vi "MT Demodulate Offset PSK.vi"(0 "input complex waveform":T4={"t0"=0.0, "dt"=1.0, "Y"=[]} {"Y" format="%.3f"; "dt" format="%^.2e"; "t0" format="%.4f"}, 5 "Offset PSK system parameters":T3={"samples per symbol (16)"=16, "symbol map"=[], "differential Offset PSK"=enum."disable"} {"symbol map" format="%.3f"}, 7 "matched filter coefficients":dbl[](array[numeric]) format="%.2f", 9 "synchronization parameters":T2 {"sync sequence" format="%.2f"}, 11 "error in (no error)":errorcluster, 12 "pulse shaping filter coefficients":dbl[](array[numeric]) format="%.2f", 13 "reset? (T)":bool=TRUE) -> (4 "recovered complex waveform":T4 {"Y" format="%.3f"; "dt" format="%^.2e"; "t0" format="%.4f"}, 6 "output bit stream":i8[](array[numeric]), 8 "measurements":T1 {"phase offset (deg)" format="%.2f"; "frequency drift (Hz)" format="%.2f"; "frequency offset (Hz)" format="%.2f"}, 10 "sync found index (symbols)":dbl format="%.4f", 15 "error out":errorcluster)   [LabVIEW 2020, in "niDMT.lvlib"]
doc: "Demodulates a offset PSK-modulated complex baseband waveform and returns the time-aligned oversampled complex waveform, the demodulated bit stream, and measurement results obtained during demodulation. This VI attempts to remove carrier and phase offset by locking to the carrier signal. \n\nNOTE: Offset mode is only supported for 4-PSK (OQPSK), and use of the offset mode requires some form of band-limiting filtration. Raised cosine and root raised cosine are the only valid filter types for OQPSK demodulation. Demodulator locking performance degrades with alpha values <0.3 in the raised cosine or root raised cosine filter design."
uses:
  <vilib>/addons/Modulation/niDMT.lvlib
  <vilib>/addons/Modulation/Analog/controls/Complex Data Waveform.ctl
  <vilib>/addons/Modulation/Digital/Support/Controls/Offset PSK System Parameters.ctl
  <vilib>/addons/Modulation/Analog/MT Resample (Complex Cluster).vi
  <vilib>/addons/Modulation/Digital/Support/Common/mod_Apply Frequency Offset (Internal).vi
  <vilib>/addons/Modulation/Analog/support/Validators/mod_Fractional Resample Validate.vi
  <vilib>/addons/Modulation/Analog/support/Validators/mod_Check Flush State.vi
  <vilib>/addons/Modulation/Analog/support/mod_FractionalResampler.vi
  <vilib>/addons/Modulation/Analog/support/mod_Integer Rate Interpolation.vi
  <vilib>/addons/Modulation/Analog/support/Validators/mod_Validate Complex Waveform.vi
  <vilib>/addons/Modulation/Analog/support/mod_PerformResampling.vi
  <vilib>/addons/Modulation/Analog/support/Validators/mod_WFErrorHandler.vi
  <vilib>/addons/Modulation/Digital/Support/Common/mod_Truncate FIR Filter (complex).vi
  <vilib>/Utility/error.llb/Error Cluster From Error Code.vi
  <vilib>/addons/Modulation/Analog/support/mod_Resampling Factors.vi
  <vilib>/addons/Modulation/Analog/support/mod_ResamplingFilter.vi
  <vilib>/addons/Modulation/Analog/support/mod_Generate Integer Interpolation Filter.vi
  <vilib>/addons/Modulation/niAMT.lvlib
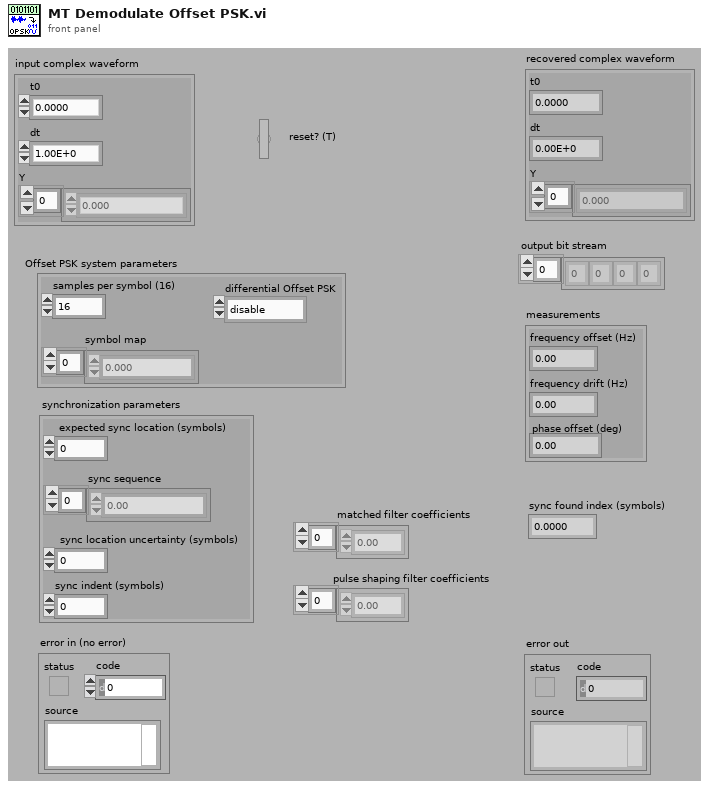
[diagram p1: front panel]
types:
  T1 = cluster{"frequency offset (Hz)":dbl, "frequency drift (Hz)":dbl, "phase offset (deg)":dbl}
  T2 = cluster{"expected sync location (symbols)":i32, "sync sequence":cdb[], "sync location uncertainty (symbols)":i32, "sync indent (symbols)":i32}
  T3 = typedef "niDMT.lvlib/Offset PSK System Parameters.ctl" = cluster{"samples per symbol (16)":i32, "symbol map":cdb[], "differential Offset PSK":enum16{"disable", "enable"}}
  T4 = typedef "niAMT.lvlib/Complex Data Waveform.ctl" = cluster{"t0":dbl, "dt":dbl, "Y":cdb[]}
  T5 = cluster{dbl, "Frequency Drift, Hz":dbl, "Phase Error Estimate, rads":dbl}
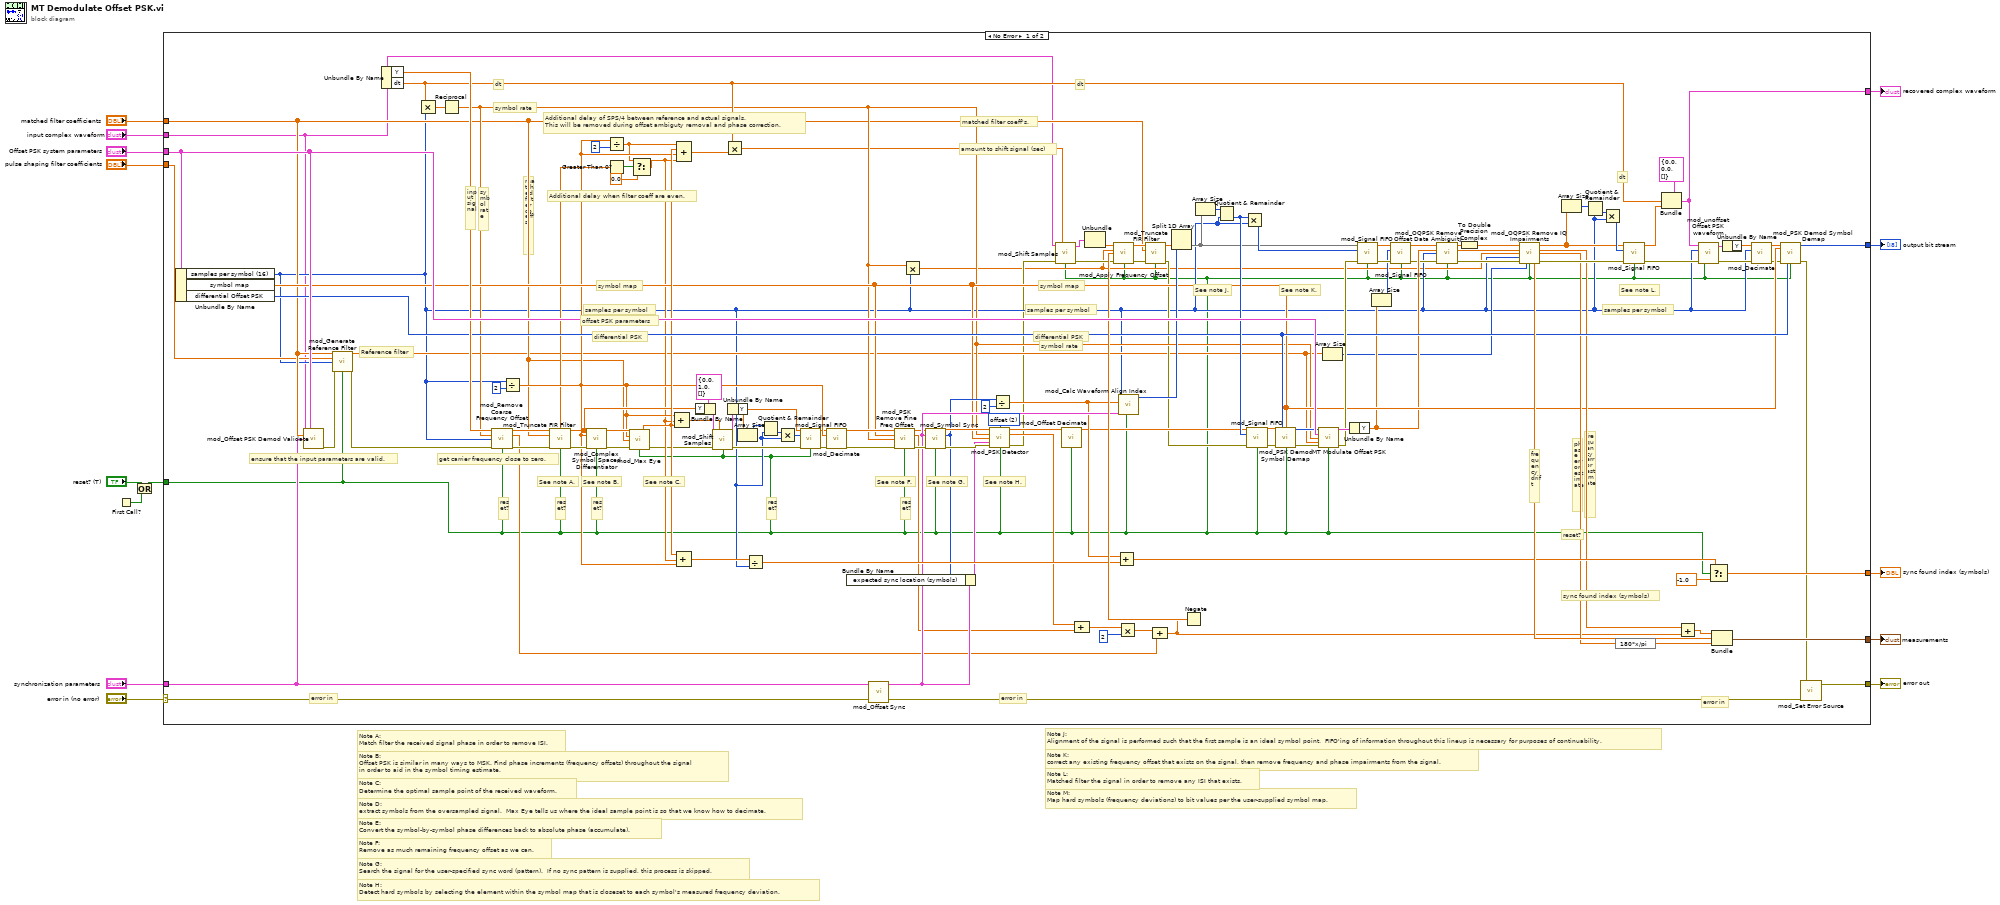
[diagram p0: block diagram]
diagram:
  # "Note E:\nConvert the symbol-by-symbol phase differences back to absolute phase (accumulate)."
  # "Note B:\nOffset PSK is similar in many ways to MSK. Find phase increments (frequency offsets) throughout the signal\nin order to aid in the symbol timing estimate."
  # "Note M:\nMap hard symbols (frequency deviations) to bit values per the user-supplied symbol map."
  # "Note J:\nAlignment of the signal is performed such that the first sample is an ideal symbol point.  FIFO'ing of information throughout this lineup is necessary for purposes of continuability."
  # "Note G:\nSearch the signal for the user-specified sync word (pattern).  If no sync pattern is supplied, this process is skipped."
  # "Note F:\nRemove as much remaining frequency offset as we can."
  # "Note D:\nextract symbols from the oversampled signal.  Max Eye tells us where the ideal sample point is so that we know how to decimate."
  # "Note C:\nDetermine the optimal sample point of the received waveform."
  # "Note A:\nMatch filter the received signal phase in order to remove ISI."
  # "Note H:\nDetect hard symbols by selecting the element within the symbol map that is closeset to each symbol's measured frequency deviation."
  # "Note K:\ncorrect any existing frequency offset that exists on the signal, then remove frequency and phase impairments from the signal."
  # "Note L:\nMatched filter the signal in order to remove any ISI that exists."
  n1 = First Call?() -> (First Call?: T/F=w5:bool)
  n2 = Or(x="reset? (T)", y=w5) -> (x .or. y?=w3:bool)
  n3 = case shown="No Error" "error in (no error)" {
    selector: "error in (no error)" -> [w136 w142]
    tunnel: w3 -> [w15 _]
    tunnel: "input complex waveform" -> [w19 _]
    tunnel: [w137 w142] -> w12
    tunnel: "matched filter coefficients" -> [w25 _]
    tunnel: [w64 _] -> w8
    tunnel: [w140 _] -> w11
    tunnel: [w89 _] -> w6
    tunnel: "Offset PSK system parameters" -> [w139 _]
    tunnel: "synchronization parameters" -> [w138 _]
    tunnel: [w141 _] -> w7
    tunnel: "pulse shaping filter coefficients" -> [w24 _]
    frame No Error {
      w54 = u16 2 items=["normal", "shifted", "offset"] ("PSK type")
      # "Additional delay when filter coeff are even."
      # "Additional delay of SPS/4 between reference and actual signals.\nThis will be removed during offset ambiguty removal and phase correction."
      # "Reference filter"
      # "samples per symbol"
      # "samples per symbol"
      # "dt"
      # "dt"
      # "dt"
      # "matched filter coeff's."
      # "symbol rate"
      # "offset PSK parameters"
      # "symbol map"
      # "symbol map"
      # "amount to shift signal (sec)"
      # "matched filter coeff's."
      # "input signal"
      # "symbol rate"
      # "differential PSK"
      # "differential PSK"
      # "samples per symbol"
      # "frequency error estimate"
      # "phase error estimate"
      # "frequency drift"
      # "reset?"
      # "sync found index (symbols)"
      # "reset?"
      # "reset?"
      # "reset?"
      # "reset?"
      # "reset?"
      # "error in"
      # "error in"
      # "error in"
      # "See note L."
      # "See note K."
      # "See note J."
      # "See note H."
      # "See note G."
      # "ensure that the input parameters are valid."
      # "See note A."
      # "See note B."
      # "get carrier frequency close to zero."
      # "See note C."
      # "See note F."
      # "symbol rate"
      n4 = Unbundle By Name(w139) -> ("samples per symbol (16)"=w22:i32, "symbol map"=w72:cdb[], "differential Offset PSK"=w86:enum16{"disable", "enable"})
      n5 = call <vilib>:"mod_Offset PSK Demod Validate.vi"("Input Complex Waveform"=w19, "PSK System Parameters"=w139, "Matched Filter Coefficients"=w25, "Synchronization Parameters"=w138) -> ("error out"=w21:errorcluster)  [unwired: 11 out]
      n6 = call <vilib>:"mod_Generate Reference Filter.vi"("matched filter coefficients"=w25, "pulse shaping filter coefficients"=w24, "samples per symbol (16)"=w22, "error in (no error)"=w21, "reset? (T)"=w15) -> ("reference filter coefficients"=w23:dbl[], "error out"=w20:errorcluster)  [unwired: 9 in]
      n7 = Unbundle By Name(w19) -> ("Y"=w113:cdb[], "dt"=w73:dbl)
      n8 = Multiply(x=w73, y=w22) -> (x*y=w134:dbl)
      n9 = Reciprocal(x=w134) -> (1/x=w71:dbl)
      n10 = call <vilib>:"mod_Remove Coarse Frequency Offset.vi"("Signal In"=w113, "Symbol Rate, Hz"=w71, "Samples Per Symbol (16)"=w22, "error in (no error)"=w20, "Reset? (T)"=w15) -> ("Signal Out"=w85:cdb[], "Freq Est, Hz"=w91:dbl, "error out"=w116:errorcluster)  [unwired: 8 out]
      n11 = Divide(x=w22, y=2) -> (x/y=w44:dbl)
      n12 = call-poly <vilib>:"mod_Truncate FIR Filter.vi"("Signal In"=w85, "Filter Coefficients"=w25, "error in (no error)"=w116, "Reset? (T)"=w15) -> ("Fractional Delay (samples)"=w41:dbl, "Signal Out"=w45:cdb[], "error out"=w115:errorcluster)  [unwired: 8 in, 1 out]
      n13 = call <vilib>:"mod_Complex Symbol Spaced Differentiator.vi"("Signal In"=w45, "Samples Per Symbol (16)"=w44, "error in (no error)"=w115, "Reset? (T)"=w15) -> ("Signal Out"=w112:cdb[], "error out"=w122:errorcluster)  [unwired: 10 out]
      n14 = Divide(x=w44, y=2) -> (x/y=w40:dbl)
      n15 = Greater Than 0?(x=w41) -> (x > 0?=w43:bool)
      n16 = call <vilib>:"mod_Max Eye.vi"("Signal In"=w112, "Samples Per Symbol (16)"=w44, "Filter Coefficients"=w25, "error in (no error)"=w122, "Reset? (T)"=w15) -> ("Waveform Alignment Offset"=w80:dbl, "error out"=w27:errorcluster)  [unwired: 6 in, 3 out]
      n17 = Select(t=w40, s=w43, f=0.0) -> (s? t:f=w39:dbl)
      n18 = Compound Arithmetic op=ADD(w44, w39, w80) -> (w28:dbl)
      n19 = Compound Arithmetic op=ADD(w80, w39, w44) -> (w114:dbl)
      n20 = Compound Arithmetic op=ADD(w40, w80, w44, w39) -> (w62:dbl)
      n21 = Bundle By Name(cluster=T4 {"t0"=0.0, "dt"=1.0, "Y"=[]} ("Input Complex Waveform"), "Y"=w45) -> (w29:T4)
      n22 = call <vilib>:"mod_Shift Samples.vi"("Input Complex Waveform"=w29, "Initial Sample Offset, sec"=w28, "error in (no error)"=w27, "Reset? (T)"=w15) -> ("Output Complex Waveform"=w30:T4, "error out"=w26:errorcluster)  [unwired: 10 in]
      n23 = Multiply(x=w73, y=w62) -> (x*y=w56:dbl)
      n24 = Unbundle By Name(w30) -> ("Y"=w37:cdb[])
      n25 = Array Size(array=w37) -> (size(s)=w34:i32)
      n26 = Divide(x=w114, y=w22) -> (x/y=w131:dbl)
      n27 = Quotient & Remainder(x=w34, y=w22) -> (floor(x/y)=w35:i32)  [unwired: 1 out]
      n28 = Multiply(x=w35, y=w22) -> (x*y=w33:i32)
      n29 = call <vilib>:"mod_Signal FIFO.vi"("Signal In"=w37, "Output Length"=w33, "error in (no error)"=w26, "Reset? (T)"=w15) -> ("Signal Out"=w32:cdb[], "error out"=w31:errorcluster)  [unwired: 10 out]
      n30 = call <vilib>:"mod_Decimate.vi"("Signal In"=w32, "Samples Per Symbol (16)"=w44, "error in (no error)"=w31) -> ("Signal Out"=w76:cdb[], "error out"=w125:errorcluster)  [unwired: 2 in, 9 out]
      n31 = call <vilib>:"mod_Offset Sync.vi"("synchronization parameters in"=w138) -> ("synchronization parameters out"=w120:T2)  [unwired: 14 out]
      n32 = call <vilib>:"mod_PSK Remove Fine Freq Offset.vi"("Symbols"=w76, "Symbol Map"=w72, "Symbol Rate, Hz"=w71, "error in (no error)"=w125, "Reset? (T)"=w15) -> ("Symbols"=w79:cdb[], "Freq Est, Hz"=w69:dbl, "error out"=w128:errorcluster)  [unwired: 8 out]
      n33 = Multiply(x=w71, y=w22) -> (x*y=w17:dbl)
      n34 = call <vilib>:"mod_Symbol Sync.vi"("Signal In"=w79, "Synchronization Parameters"=w120, "error in (no error)"=w128, "Reset? (T)"=w15) -> ("Signal Out"=w127:cdb[], "Sync Location (symbols)"=w119:i32, "error out"=w126:errorcluster)  [unwired: 9 out]
      n35 = Bundle By Name(cluster=w120, "expected sync location (symbols)"=w119) -> (w124:T2)
      n36 = call <vilib>:"mod_PSK Detector.vi"("Signal In"=w127, "PSK type"=w54, "Symbol Rate, Hz"=w71, "Symbol Map"=w72, "Synchronization Parameters"=w124, "error in (no error)"=w126, "Reset (T)"=w15) -> ("Signal Out"=w75:cdb[], "Freq Est, Hz"=w68:dbl, "error out"=w18:errorcluster)  [unwired: 5 in, 1 out]
      n37 = Divide(x=w119, y=2) -> (x/y=w117:dbl)
      n38 = call <vilib>:"mod_Shift Samples.vi"("Input Complex Waveform"=w19, "Initial Sample Offset, sec"=w56, "error in (no error)"=w18, "Reset? (T)"=w15) -> ("Output Complex Waveform"=w55:T4, "error out"=w111:errorcluster)  [unwired: 10 in]
      n39 = call <vilib>:"mod_Offset Decimate.vi"("Symbols In"=w75, "Reset (T)"=w15) -> ("Symbols Out"=w83:cdb[])  [unwired: 13 out]
      n40 = Compound Arithmetic op=ADD(w68, w69) -> (w67:dbl)
      n41 = Unbundle(w55) -> ("Y"=w78:cdb[])  [unwired: 2 out]
      n42 = Add(x=w117, y=w131) -> (x+y=w108:dbl)
      n43 = Multiply(x=w67, y=2) -> (x*y=w70:dbl)
      n44 = call <vilib>:"mod_Calc Waveform Align Index.vi"("Reset? (T)"=w15, "Synchronization Parameters"=w120, "Sync Location, symbols"=w117, "Samples Per Symbol (16)"=w22) -> ("align index, samples"=w105:i32)  [unwired: 7 out]
      n45 = Compound Arithmetic op=ADD(w70, w91) -> (w63:dbl)
      n46 = Negate(x=w63) -> (-x=w135:dbl)
      n47 = call <vilib>:"mod_Apply Frequency Offset.vi"("Signal In"=w78, "Rate, pts/sec"=w17, "Freq Offset, Hz"=w135, "error in (no error)"=w111, "Reset? (T)"=w15) -> ("Signal Out"=w84:cdb[], "error out"=w47:errorcluster)  [unwired: 9 out]
      n48 = call-poly <vilib>:"mod_Truncate FIR Filter.vi"("Signal In"=w84, "Filter Coefficients"=w25, "error in (no error)"=w47, "Reset? (T)"=w15) -> ("Signal Out"=w74:cdb[], "error out"=w46:errorcluster)  [unwired: 8 in, 2 out]
      n49 = Split 1D Array(array=w74, index=w105) -> (second subarray=w77:cdb[])  [unwired: 1 out]
      n50 = Array Size(array=w77) -> (size(s)=w106:i32)
      n51 = Quotient & Remainder(x=w106, y=w22) -> (floor(x/y)=w103:i32)  [unwired: 1 out]
      n52 = Multiply(x=w103, y=w22) -> (x*y=w104:i32)
      n53 = call <vilib>:"mod_Signal FIFO.vi"("Signal In"=w83, "Output Length"=w103, "error in (no error)"=w46, "Reset? (T)"=w15) -> ("Signal Out"=w93:cdb[], "error out"=w107:errorcluster)  [unwired: 10 out]
      n54 = call <vilib>:"mod_PSK Demod Symbol Demap.vi"("Symbols In"=w93, "Differential PSK Enable"=w86, "Symbol Map"=w72, "error in (no error)"=w107, "Reset? (T)"=w15) -> ("Bits Out"=w92:i8[], "error out"=w121:errorcluster)  [unwired: 9 out]
      n55 = call <vilib>:"MT Modulate Offset PSK.vi"("input bit stream"=w92, "Offset PSK system parameters"=w139, "symbol rate (Hz)"=w71, "pulse shaping filter coefficients"=w23, "error in (no error)"=w121, "reset? (T)"=w15) -> ("output complex waveform"=w132:T4, "error out"=w95:errorcluster)  [unwired: 1 in, 7 out]
      n56 = Array Size(array=w23) -> (size(s)=w36:i32)
      n57 = Unbundle By Name(w132) -> ("Y"=w66:cdb[])
      n58 = call <vilib>:"mod_Signal FIFO.vi"("Signal In"=w77, "Output Length"=w104, "error in (no error)"=w95, "Reset? (T)"=w15) -> ("Signal Out"=w101:cdb[], "error out"=w102:errorcluster)  [unwired: 10 out]
      n59 = Array Size(array=w66) -> (size(s)=w100:i32)
      n60 = call <vilib>:"mod_Signal FIFO.vi"("Signal In"=w101, "Output Length"=w100, "error in (no error)"=w102, "Reset? (T)"=w15) -> ("Signal Out"=w61:cdb[], "error out"=w65:errorcluster)  [unwired: 10 out]
      n61 = call <vilib>:"mod_OQPSK Remove Offset Data Ambiguity.vi"("Received Signal In"=w61, "Reference Signal"=w66, "Samples Per Symbol"=w22, "error in (no error)"=w65, "Reset? (T)"=w15) -> ("Received Signal Out"=w60:cdb[], "Reference Signal Out"=w59:cdb[], "error out"=w94:errorcluster)  [unwired: 8 in]
      n62 = To Double Precision Complex(1:w60) -> (0:w57:cdb[])
      n63 = call <vilib>:"mod_OQPSK Remove IQ Impairments.vi"("Received Signal In"=w57, "Reference Signal"=w59, "Signal Rate, Hz"=w17, "Sample per Symbol"=w22, "error in (no error)"=w94, "Filter Length (Samples)"=w36, "Reset?"=w15) -> ("Received Signal Out"=w58:cdb[], "Frequency Estimate, Hz"=w82:dbl, "Phase Error Estimate, rads"=w81:dbl, "Frequency Drift, Hz"=w130:dbl, "error out"=w99:errorcluster)  [unwired: 3 in, 1 out]
      n64 = Array Size(array=w58) -> (size(s)=w98:i32)
      n65 = Quotient & Remainder(x=w98, y=w22) -> (floor(x/y)=w97:i32)  [unwired: 1 out]
      n66 = Multiply(x=w97, y=w22) -> (x*y=w96:i32)
      n67 = expression code="180*x/pi"(w81) -> (w16:dbl)
      n68 = call <vilib>:"mod_Signal FIFO.vi"("Signal In"=w58, "Output Length"=w96, "error in (no error)"=w99, "Reset? (T)"=w15) -> ("Signal Out"=w53:cdb[], "error out"=w51:errorcluster)  [unwired: 10 out]
      n69 = Bundle(cluster=T4 {"t0"=0.0, "dt"=0.0, "Y"=[]} ("Recovered Complex Waveform"), "dt"=w73, "Y"=w53) -> (w89:T4)  [unwired: 1 out]
      n70 = Add(x=w82, y=w63) -> (x+y=w90:dbl)
      n71 = call <vilib>:"mod_unoffset Offset PSK waveform.vi"("input complex waveform"=w89, "samples per symbol (16)"=w22, "error in (no error)"=w51, "reset? (T)"=w15) -> ("output complex waveform"=w88:T4, "error out"=w50:errorcluster)  [unwired: 10 out]
      n72 = Select(t=w108, s=w15, f=-1.0) -> (s? t:f=w140:dbl)
      n73 = Bundle(w90, "Frequency Drift, Hz"=w130, "Phase Error Estimate, rads"=w16) -> (w141:T5)  [unwired: 1 out]
      n74 = Unbundle By Name(w88) -> ("Y"=w52:cdb[])
      n75 = call <vilib>:"mod_Decimate.vi"("Signal In"=w52, "Samples Per Symbol (16)"=w22, "error in (no error)"=w50) -> ("Signal Out"=w87:cdb[], "error out"=w49:errorcluster)  [unwired: 2 in, 9 out]
      n76 = call <vilib>:"mod_PSK Demod Symbol Demap.vi"("Symbols In"=w87, "Differential PSK Enable"=w86, "Symbol Map"=w72, "error in (no error)"=w49, "Reset? (T)"=w15) -> ("Bits Out"=w64:i8[], "error out"=w48:errorcluster)  [unwired: 9 out]
      n77 = call <vilib>:"mod_Set Error Source.vi"("initial error in (no error)"=w136, "final error in (no error)"=w48) -> ("error out"=w137:errorcluster)  [unwired: 3 out]
    }
    frame Error {
    }
  }
  "error out" <- w12
  "sync found index (symbols)" <- w11
  "output bit stream" <- w8
  "recovered complex waveform" <- w6
  "measurements" <- w7
